vi "Refresh Hierarchy View - Populate Table.vi"(8 "error in (no error)":errorcluster, 10 "BOM Items Raw Data":T1[](array[typedef]), 11 "TreeControl in":refnum<vi>) -> (0 "error out":errorcluster)   [LabVIEW 2018]
uses:
  TypeDef/BOM Table Raw Items.ctl
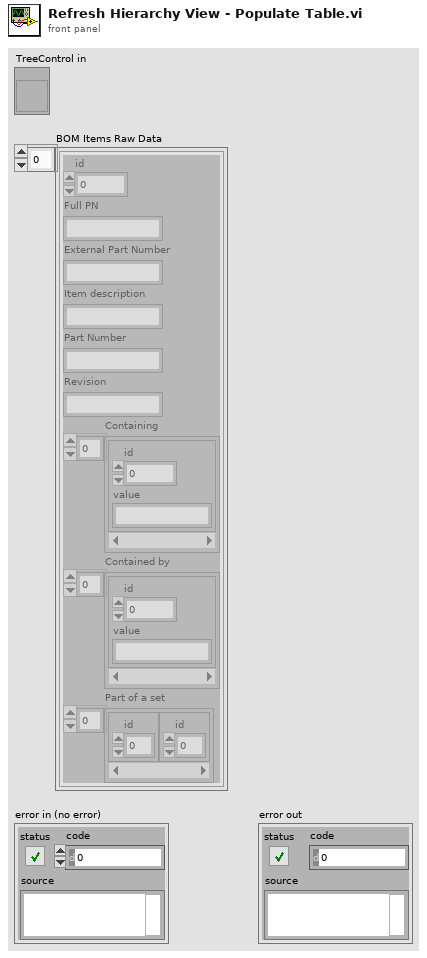
[diagram p1: front panel]
types:
  T1 = typedef "BOM Table Raw Items.ctl" = cluster{"id":i32, "Full PN":string, "External Part Number":string, "Item description":string, "Part Number":string, "Revision":string, "Containing":cluster{"id":i32, "value":string}[], "Contained by":cluster{"id":i32, "value":string}[], "Part of a set":cluster{"id":i32}[]}
  T2 = cluster{"ID":i32, "Item":cluster{"id":i32}[], "Contains":cluster{"id":i32}[], "Amount of Times":string, "Length (mm)":string}
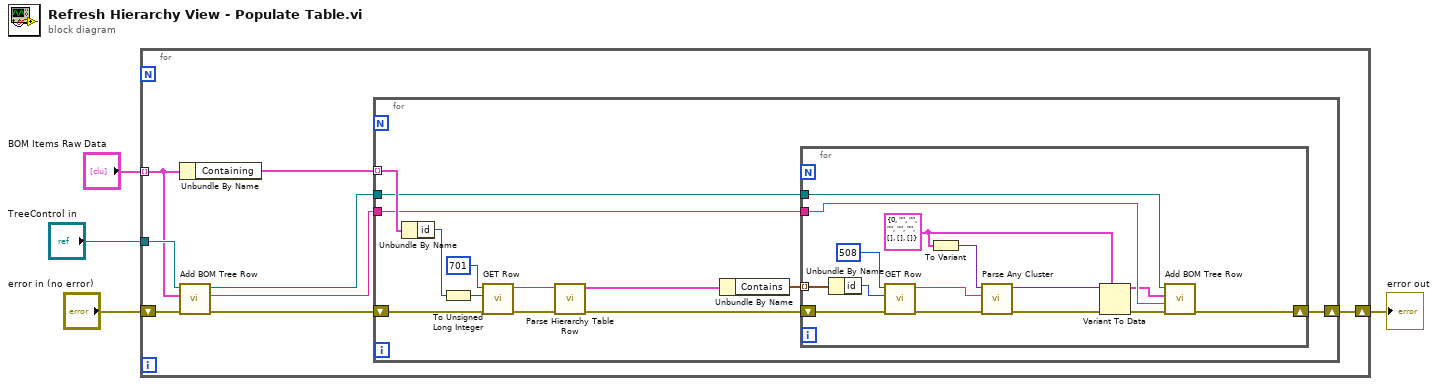
[diagram p0: block diagram]
diagram:
  n1 = for {
    tunnel: "TreeControl in" -> [w11]
    shift-right: [w9] -> w2
    shift-left: "error in (no error)" -> [w12]
    tunnel: "BOM Items Raw Data" -> [w6] mode=indexing
    n2 = Unbundle By Name(w6) -> ("Containing"=w5:cluster{"id":i32, "value":string}[])
    n3 = call "Add BOM Tree Row.vi"("error in (no error)"=w12, "BOM Table Raw Items"=w6, "TreeControl in"=w11) -> ("error out"=w10:errorcluster, "New Item Tag"=w7:string, "TreeControl out"=w8:refnum<vi>)  [unwired: 6 in]
    n4 = for {
      shift-right: [w15] -> w9
      shift-left: w10 -> [w18]
      tunnel: w5 -> [w24] mode=indexing
      tunnel: w8 -> [w17]
      tunnel: w7 -> [w16]
      n5 = Unbundle By Name(w24) -> ("id"=w14:i32)
      n6 = To Unsigned Long Integer(number=w14) -> (unsigned 32bit integer=w13:u32)
      n7 = call "GET Row.vi"("Error in"=w18, "Row ID"=w13, "Table ID"=u32 701) -> ("Error out"=w22:errorcluster, "Rows Array JSON"=w23:string)  [unwired: 7 in]
      n8 = call "Parse Hierarchy Table Row.vi"("Error in"=w22, "Rows Array JSON"=w23) -> ("Error out"=w19:errorcluster, "data"=w21:T2)  [unwired: 8 in]
      n9 = Unbundle By Name(w21) -> ("Contains"=w20:cluster{"id":i32}[])
      n10 = for {
        tunnel: w20 -> [w40] mode=indexing
        shift-right: [w27] -> w15
        shift-left: w19 -> [w37]
        tunnel: w17 -> [w36]
        tunnel: w16 -> [w35]
        w34 = T1 {"id"=0, "Full PN"="", "External Part Number"="", "Item description"="", "Part Number"="", "Revision"="", "Containing"=[], "Contained by"=[], "Part of a set"=[]}
        n11 = Unbundle By Name(w40) -> ("id"=w39:i32)
        n12 = call "GET Row.vi"("Error in"=w37, "Row ID"=w39, "Table ID"=u32 508) -> ("Error out"=w30:errorcluster, "Rows Array JSON"=w33:string)  [unwired: 7 in]
        n13 = To Variant(anything=w34) -> (Variant=w32:variant)
        n14 = call "Parse Any Cluster.vi"("error in (no error)"=w30, "JSON In"=w33, "Cluster in"=w32) -> ("error out"=w26:errorcluster, "Cluster out"=w31:variant)  [unwired: 7 in]
        n15 = Variant To Data(error in=w26, type=w34, Variant=w31) -> (data=w29:T1, error out=w28:errorcluster)
        n16 = call "Add BOM Tree Row.vi"("error in (no error)"=w28, "Parent Tag"=w35, "BOM Table Raw Items"=w29, "TreeControl in"=w36) -> ("error out"=w27:errorcluster)  [unwired: 5 in, 2 out]
      }
    }
  }
  "error out" <- w2
